vi "Create Serial Output Channel CSI-2 IO x2.vi"() -> (4 "serial output channel csi-2 io x2":T4)   [LabVIEW 2020, in "GettingStarted_Common_148X_FPGA.lvlib"]
uses:
  GettingStarted_Common_148X_FPGA.lvlib
  Types/Serial Output Channel IO.ctl
  Types/Serial Output Channel IO 32b.ctl
  Types/Serial Output Channel IO 64b.ctl
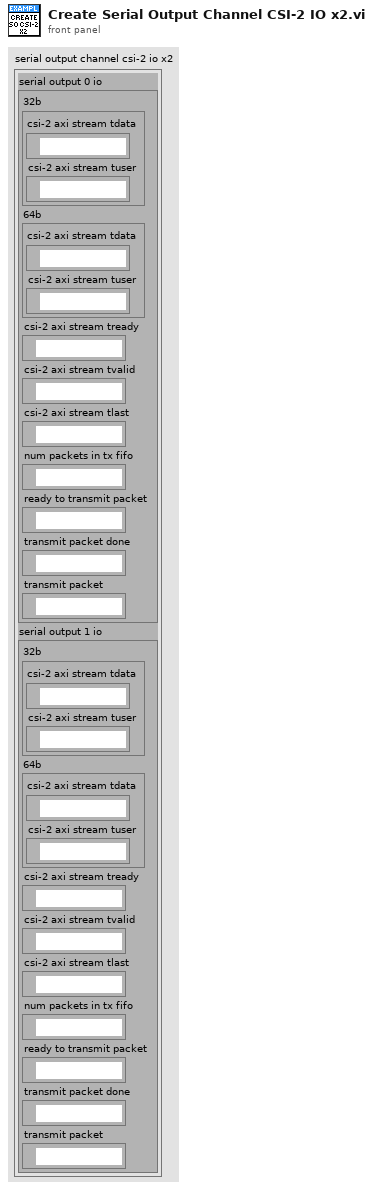
[diagram p1: front panel]
types:
  T1 = typedef "GettingStarted_Common_148X_FPGA.lvlib/Serial Output Channel IO.ctl" = cluster{"32b":T2, "64b":T3, "csi-2 axi stream tready":refnum<k21>, "csi-2 axi stream tvalid":refnum<k21>, "csi-2 axi stream tlast":refnum<k21>, "num packets in tx fifo":refnum<k21>, "ready to transmit packet":refnum<k21>, "transmit packet done":refnum<k21>, "transmit packet":refnum<k21>}
  T2 = typedef "GettingStarted_Common_148X_FPGA.lvlib/Serial Output Channel IO 32b.ctl" = cluster{"csi-2 axi stream tdata":refnum<k21>, "csi-2 axi stream tuser":refnum<k21>}
  T3 = typedef "GettingStarted_Common_148X_FPGA.lvlib/Serial Output Channel IO 64b.ctl" = cluster{"csi-2 axi stream tdata":refnum<k21>, "csi-2 axi stream tuser":refnum<k21>}
  T4 = cluster{"serial output 0 io":T1, "serial output 1 io":T1}
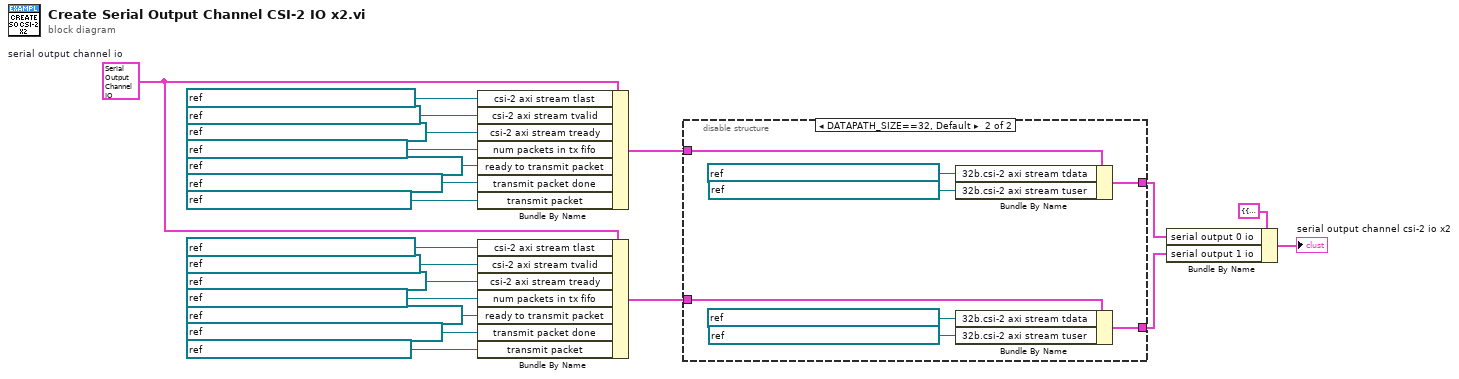
[diagram p0: block diagram]
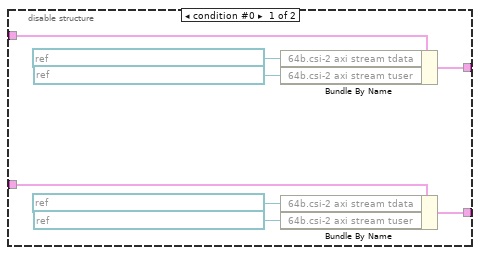
[diagram p2: hidden frame]
diagram:
  w6 = T1 {"32b"={"csi-2 axi stream tdata"="", "csi-2 axi stream tuser"=""}, "64b"={"csi-2 axi stream tdata"="", "csi-2 axi stream tuser"=""}, "csi-2 axi stream tready"="", "csi-2 axi stream tvalid"="", "csi-2 axi stream tlast"="", "num packets in tx fifo"="", "ready to transmit packet"="", "transmit packet done"="", "transmit packet"=""}  # serial output channel io
  n1 = Bundle By Name(cluster=w6, "csi-2 axi stream tlast"=refnum<k21> "IO Socket\\SO 0 CSI-2 AXI Stream TLast", "csi-2 axi stream tvalid"=refnum<k21> "IO Socket\\SO 0 CSI-2 AXI Stream TValid", "csi-2 axi stream tready"=refnum<k21> "IO Socket\\SO 0 CSI-2 AXI Stream TReady", "num packets in tx fifo"=refnum<k21> "IO Socket\\SO 0 CSI-2 Packets In FIFO", "ready to transmit packet"=refnum<k21> "IO Socket\\SO 0 CSI-2 Ready To Transmit Packet", "transmit packet done"=refnum<k21> "IO Socket\\SO 0 CSI-2 Transmit Packet Done", "transmit packet"=refnum<k21> "IO Socket\\SO 0 CSI-2 Transmit Packet") -> (w4:T1)
  n2 = Bundle By Name(cluster=w6, "csi-2 axi stream tlast"=refnum<k21> "IO Socket\\SO 1 CSI-2 AXI Stream TLast", "csi-2 axi stream tvalid"=refnum<k21> "IO Socket\\SO 1 CSI-2 AXI Stream TValid", "csi-2 axi stream tready"=refnum<k21> "IO Socket\\SO 1 CSI-2 AXI Stream TReady", "num packets in tx fifo"=refnum<k21> "IO Socket\\SO 1 CSI-2 Packets In FIFO", "ready to transmit packet"=refnum<k21> "IO Socket\\SO 1 CSI-2 Ready To Transmit Packet", "transmit packet done"=refnum<k21> "IO Socket\\SO 1 CSI-2 Transmit Packet Done", "transmit packet"=refnum<k21> "IO Socket\\SO 1 CSI-2 Transmit Packet") -> (w3:T1)
  n3 = disable-structure shown="DATAPATH_SIZE==32, Default" {
    disable-tunnel: [w22 w34] -> w2
    disable-tunnel: [w23 w35] -> w1
    disable-tunnel: w4 -> [w27 w37]
    disable-tunnel: w3 -> [w26 w36]
    frame condition #0 {
      n4 = Bundle By Name(cluster=w27, "64b.csi-2 axi stream tdata"=refnum<k21> "IO Socket\\SO 0 CSI-2 AXI Stream TData" ("csi-2 axi stream tdata"), "64b.csi-2 axi stream tuser"=refnum<k21> "IO Socket\\SO 0 CSI-2 AXI Stream TUser" ("csi-2 axi stream tuser")) -> (w22:T1)
      n5 = Bundle By Name(cluster=w26, "64b.csi-2 axi stream tdata"=refnum<k21> "IO Socket\\SO 1 CSI-2 AXI Stream TData" ("csi-2 axi stream tdata"), "64b.csi-2 axi stream tuser"=refnum<k21> "IO Socket\\SO 1 CSI-2 AXI Stream TUser" ("csi-2 axi stream tuser")) -> (w23:T1)
    }
    frame condition #1 (active) {
      n6 = Bundle By Name(cluster=w37, "32b.csi-2 axi stream tdata"=refnum<k21> "IO Socket\\SO 0 CSI-2 AXI Stream TData" ("csi-2 axi stream tdata"), "32b.csi-2 axi stream tuser"=refnum<k21> "IO Socket\\SO 0 CSI-2 AXI Stream TUser" ("csi-2 axi stream tuser")) -> (w34:T1)
      n7 = Bundle By Name(cluster=w36, "32b.csi-2 axi stream tdata"=refnum<k21> "IO Socket\\SO 1 CSI-2 AXI Stream TData" ("csi-2 axi stream tdata"), "32b.csi-2 axi stream tuser"=refnum<k21> "IO Socket\\SO 1 CSI-2 AXI Stream TUser" ("csi-2 axi stream tuser")) -> (w35:T1)
    }
  }
  n8 = Bundle By Name(cluster=T4 {"serial output 0 io"={"32b"={"csi-2 axi stream tdata"="", "csi-2 axi stream tuser"=""}, "64b"={"csi-2 axi stream tdata"="", "csi-2 axi stream tuser"=""}, "csi-2 axi stream tready"="", "csi-2 axi stream tvalid"="", "csi-2 axi stream tlast"="", "num packets in tx fifo"="", "ready to transmit packet"="", "transmit packet done"="", "transmit packet"=""}, "serial output 1 io"={"32b"={"csi-2 axi stream tdata"="", "csi-2 axi stream tuser"=""}, "64b"={"csi-2 axi stream tdata"="", "csi-2 axi stream tuser"=""}, "csi-2 axi stream tready"="", "csi-2 axi stream tvalid"="", "csi-2 axi stream tlast"="", "num packets in tx fifo"="", "ready to transmit packet"="", "transmit packet done"="", "transmit packet"=""}} ("serial output channel csi-2 io x4"), "serial output 0 io"=w2, "serial output 1 io"=w1) -> (→"serial output channel csi-2 io x2":T4)
